vi "NewCustomVIOwnerByUID.vi"(4 "path":path, 5 "vi object class":refnum<vi>, 6 "location":T1, 8 "error in (no error)":errorcluster, 10 "owner":cluster{"owner?":bool, "ownerUID":i32}, 11 "targetVI":refnum<vi>) -> (0 "error out":errorcluster, 1 "UID":i32, 2 "object refnum":refnum<vi>, 3 "dup targetVI":refnum<vi>)   [LabVIEW 2013]
uses:
  <vilib>/Utility/miscctls.llb/LVPointTypeDef.ctl
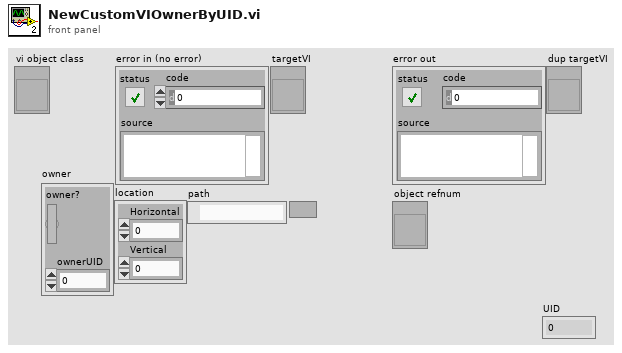
[diagram p1: front panel]
types:
  T1 = typedef "LVPointTypeDef.ctl" = cluster{"Horizontal":i16, "Vertical":i16}
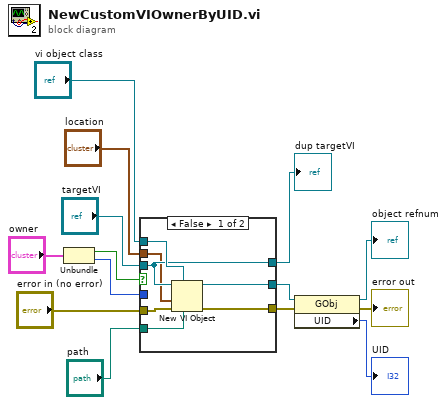
[diagram p0: block diagram]
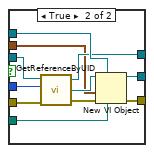
[diagram p2: hidden frame]
diagram:
  n1 = Unbundle("owner") -> ("owner?"=w14:bool, "ownerUID"=w13:i32)
  n2 = case shown="False" w14 {
    tunnel: "error in (no error)" -> [w20 w31]
    tunnel: "targetVI" -> [w17 w32]
    tunnel: w13 -> [_ w30]
    tunnel: [w21 w24] -> w3
    tunnel: [w19 w28] -> w6
    tunnel: "vi object class" -> [w18 w27]
    tunnel: [w17 w25] -> w7
    tunnel: "location" -> [w16 w23]
    tunnel: "path" -> [w15 w22]
    frame False {
      n3 = New VI Object(vi object class=w18, owner refnum=w17, position/next to=w16, 6:w15, 8:w20) -> (object refnum=w19:refnum<vi>, 0:w21:errorcluster)  [unwired: 3 in]
    }
    frame True {
      n4 = call "GetReferenceByUID.vi"("error in (no error)"=w31, "UID"=w30, "targetVI"=w32) -> ("error out"=w29:errorcluster, "refNum"=w26:refnum<vi>, "dup targetVI"=w25:refnum<vi>)  [unwired: 1 in]
      n5 = New VI Object(vi object class=w27, owner refnum=w26, position/next to=w23, 6:w22, 8:w29) -> (object refnum=w28:refnum<vi>, 0:w24:errorcluster)  [unwired: 3 in]
    }
  }
  "dup targetVI" <- w7
  n6 = property class="GObj"(reference=w6, error in=w3) -> (reference out=→"object refnum":refnum<vi>, error out=→"error out":errorcluster, "UID"=→"UID":i32)
